vi "CleanUp.vi"(8 "Error In":errorcluster, 11 "Object in":refnum<class "Snake.lvclass">) -> (0 "Error Out":errorcluster, 3 "object out":refnum<class "Snake.lvclass">)   [LabVIEW 2021, in "Snake.lvclass"]
uses:
  Snake.lvclass
  Snake.lvclass/Snake.ctl
  GameEl_class/GameEl.lvclass
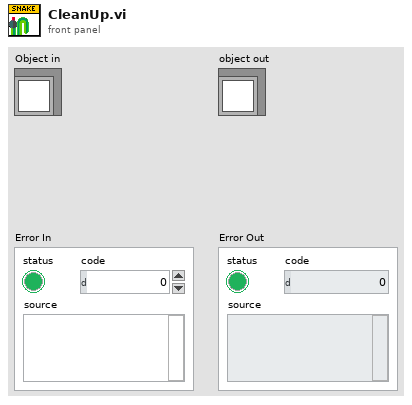
[diagram p1: front panel]
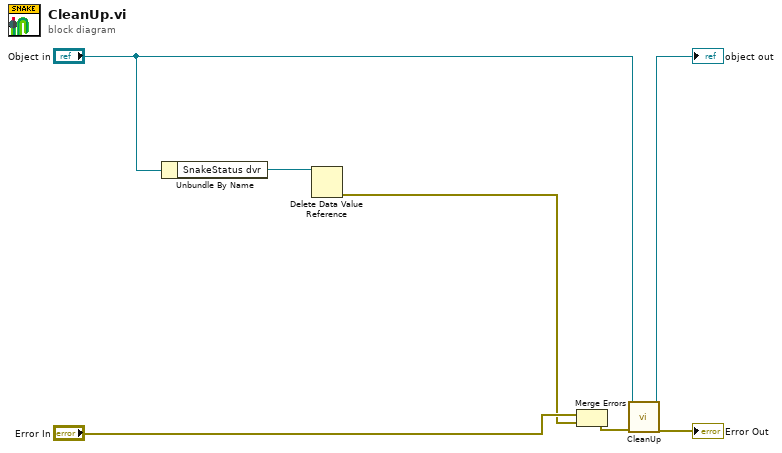
[diagram p0: block diagram]
diagram:
  n1 = Unbundle By Name("Object in") -> ("SnakeStatus dvr"=w2:refnum<data-value>)
  n2 = Delete Data Value Reference(data value reference=w2) -> (error out=w1:errorcluster)  [unwired: 1 in, 1 out]
  n3 = Merge Errors("Error In", w1) -> (w5:errorcluster)
  n4 = call-parent "CleanUp.vi"("Error In"=w5, "object in"="Object in") -> ("Error Out"=→"Error Out":errorcluster, "object out"=→"object out":refnum<class "Snake.lvclass">)  [unwired: 8 in]
